vi "take_data.vi"(9 "data stage":bool, 10 "phase stage":bool, 11 "iteration":dbl) -> (3 "take data":bool)   [LabVIEW 2015]
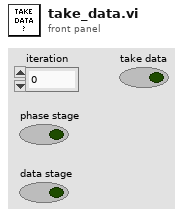
[diagram p1: front panel]
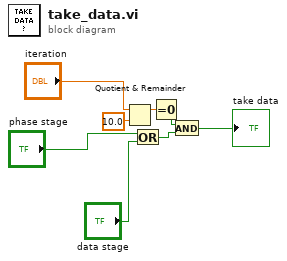
[diagram p0: block diagram]
diagram:
  n1 = Quotient & Remainder(x="iteration", y=10.0) -> (x-y*floor(x/y)=w8:dbl)  [unwired: 1 out]
  n2 = Or(x="phase stage", y="data stage") -> (x .or. y?=w4:bool)
  n3 = Equal To 0?(x=w8) -> (x = 0?=w3:bool)
  n4 = And(x=w3, y=w4) -> (x .and. y?=→"take data":bool)
